vi "Periodic Tasks.vi"(8 "error in":errorcluster) -> ()   [LabVIEW 2018]
doc: "This VI runs in parallel to other tasks. It can contain as many user-defined periodic loops as you need. These can carry out PID or other sorts of timed response."
uses:
  Classes/Vision/PublicMethods/FilteredVisionData.ctl
  Classes/Vision/Vision.lvclass
  RobotGlobal.vi
panel:
  in  "FilteredVisionData 6":T1
  in  "FilteredVisionData 5":T1
  in  "FilteredVisionData 4":T1
  in  "FilteredVisionData 3":T1
  in  "FilteredVisionData 2":T1
  in  "FilteredVisionData":T1
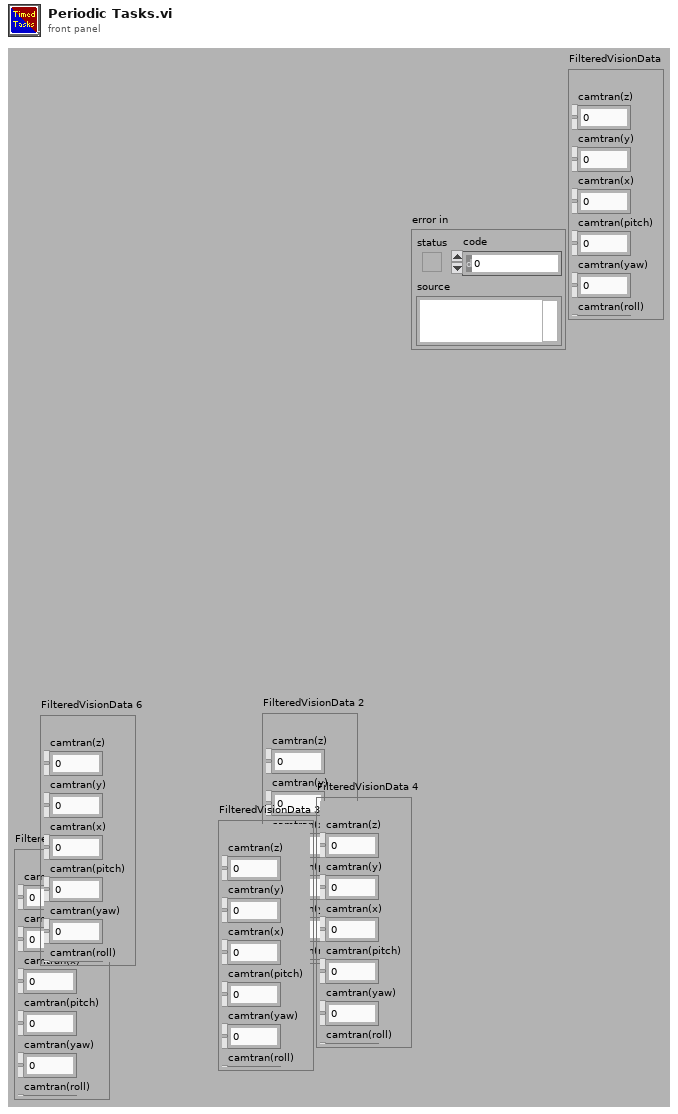
[diagram p1: front panel]
types:
  T1 = typedef "Vision.lvlib/Vision.lvclass/FilteredVisionData.ctl" = cluster{"camtran(z)":dbl, "camtran(x)":dbl, "camtran(pitch)":dbl, "camtran(y)":dbl, "camtran(roll)":dbl, "camtran(yaw)":dbl}
  T2 = typedef "RobotObjects.ctl" = cluster{"Drive.lvclass":refnum<class "Drive.lvclass">, "Pneumatics.lvclass":refnum<class "Pneumatics.lvclass">, "Vision.lvclass":refnum<class "Vision.lvclass">, "Joysticks.lvclass":refnum<class "Joysticks.lvclass">, "Elevator.lvclass":refnum<class "Elevator.lvclass">, "Hatch.lvclass":refnum<class "Hatch.lvclass">, "Cargo.lvclass":refnum<class "Cargo.lvclass">}
  T3 = typedef "Vision.lvlib/Vision.lvclass/LimeLightData.ctl" = cluster{"Target?(tv)":dbl, "HorOffset(tx)":dbl, "VertOffset(ty)":dbl, "TargetArea(ta)":dbl, "Skew/roll(ts)":dbl, "PipelinLatency(tl)":dbl, "Sidelength of shortest side of the fitted bounding box (tshort) ":dbl, "Sidelength of longest side of the fitted bounding box (tlong)":dbl, "Horizontal sidelength of the rough bounding box (thor)":dbl, "Vertical sidelength of the rough bounding box (tvert)":dbl, "Pipeline?(GetPipe)":dbl, "camtran(x)":dbl, "camtran(y)":dbl, "camtran(z)":dbl, "camtran(pitch)":dbl, "camtran(yaw)":dbl, "camtran(roll)":dbl}
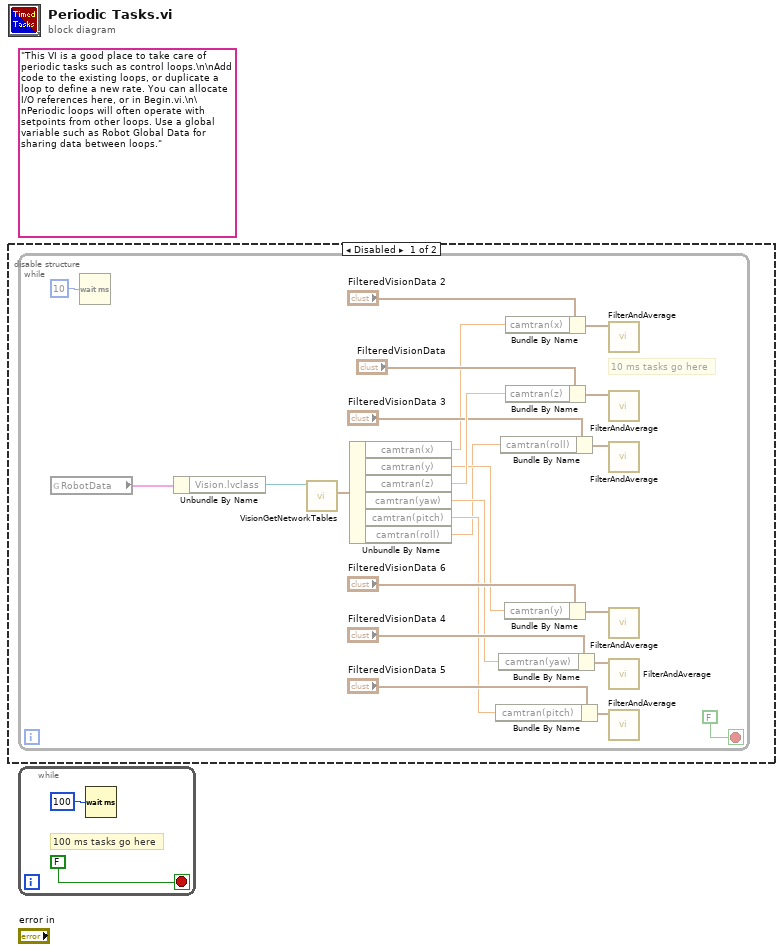
[diagram p0: block diagram]
diagram:
  (unwired) "This VI is a good place to take care of periodic tasks such as control loops.\n\nAdd code to the existing loops, or duplicate a loop to define a new rate. You can allocate I/O references here, or in Begin.vi.\n\nPeriodic loops will often operate with setpoints from other loops. Use a global variable such as Robot Global Data for sharing data between loops."
  n1 = disable-structure shown="Disabled" {
    frame Disabled {
      n2 = while {
        stop <- FALSE stop-if-true
        # "10 ms tasks go here"
        n3 = global read "RobotGlobal.vi" "RobotData"() -> (w20:T2)
        n4 = Wait (ms)(milliseconds to wait=u32 10) -> ()  [unwired: 1 out]
        n5 = Unbundle By Name(w20) -> ("Vision.lvclass"=w21:refnum<class "Vision.lvclass">)
        n6 = call "VisionGetNetworkTables.vi"("Vision in"=w21) -> ("Cluster"=w19:T3)  [unwired: 8 in, 2 out]
        n7 = Unbundle By Name(w19) -> ("camtran(x)"=w5:dbl, "camtran(y)"=w4:dbl, "camtran(z)"=w18:dbl, "camtran(yaw)"=w3:dbl, "camtran(pitch)"=w2:dbl, "camtran(roll)"=w1:dbl)
        n8 = Bundle By Name(cluster="FilteredVisionData 5", "camtran(pitch)"=w2) -> (w8:T1)
        n9 = Bundle By Name(cluster="FilteredVisionData 4", "camtran(yaw)"=w3) -> (w10:T1)
        n10 = Bundle By Name(cluster="FilteredVisionData 3", "camtran(roll)"=w1) -> (w12:T1)
        n11 = Bundle By Name(cluster="FilteredVisionData 6", "camtran(y)"=w4) -> (w6:T1)
        n12 = Bundle By Name(cluster="FilteredVisionData 2", "camtran(x)"=w5) -> (w14:T1)
        n13 = Bundle By Name(cluster="FilteredVisionData", "camtran(z)"=w18) -> (w16:T1)
        n14 = call "FilterAndAverage.vi"("FilteredVisionData"=w14) -> ()  [unwired: 10 in, 1 out]
        n15 = call "FilterAndAverage.vi"("FilteredVisionData"=w16) -> ()  [unwired: 10 in, 1 out]
        n16 = call "FilterAndAverage.vi"("FilteredVisionData"=w12) -> ()  [unwired: 10 in, 1 out]
        n17 = call "FilterAndAverage.vi"("FilteredVisionData"=w6) -> ()  [unwired: 10 in, 1 out]
        n18 = call "FilterAndAverage.vi"("FilteredVisionData"=w10) -> ()  [unwired: 10 in, 1 out]
        n19 = call "FilterAndAverage.vi"("FilteredVisionData"=w8) -> ()  [unwired: 10 in, 1 out]
      }
    }
    frame Enabled {
    }
  }
  n20 = while {
    stop <- FALSE stop-if-true
    # "100 ms tasks go here"
    n21 = Wait (ms)(milliseconds to wait=u32 100) -> ()  [unwired: 1 out]
  }
